vi "Try fsync.vi"(6 "Deadline in":T2, 8 "error in (no error)":errorcluster, 10 "handle":T1 format="%02x", 11 "session in":refnum<class "Session.lvclass">) -> (0 "error out":errorcluster, 3 "session out":refnum<class "Session.lvclass">)   [LabVIEW 2020, in "NI_SFTP.lvlib"]
uses:
  <vilib>/net/SFTP/NI_SFTP.lvlib
  <vilib>/Utility/Deadline/Deadline.ctl
  <vilib>/Utility/Deadline/Mode.ctl
  <vilib>/net/SFTP/Session/Session.lvclass
  <vilib>/net/SFTP/Session/Handle.ctl
  <vilib>/net/SFTP/API/Support/Command/fsync_openssh.com/fsync_openssh.com.lvclass
  <vilib>/Utility/Deadline/NI_Deadline.lvlib
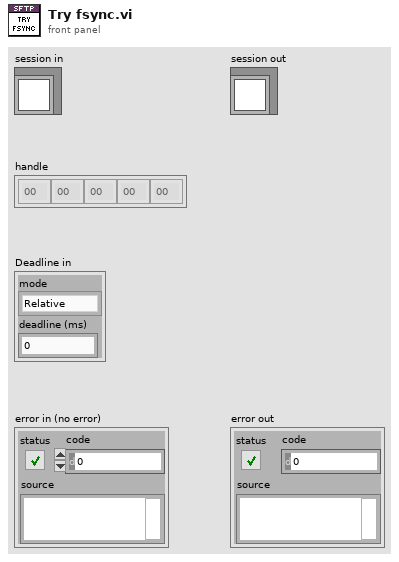
[diagram p1: front panel]
types:
  T1 = typedef "NI_SFTP.lvlib/Session.lvclass/Handle.ctl" = u8[]
  T2 = typedef "NI_Deadline.lvlib/Deadline.ctl" = cluster{"mode":T3, "deadline (ms)":u32}
  T3 = typedef "NI_Deadline.lvlib/Mode.ctl" = enum16{"Relative", "Use deadline", "Wait forever", "Nonblocking", "N/A"}
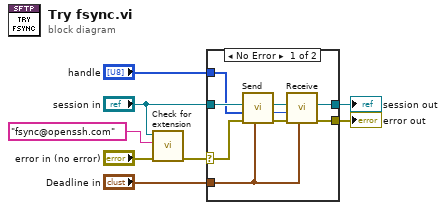
[diagram p0: block diagram]
diagram:
  n1 = call <vilib>:"Check for extension.vi"("error in (no error)"="error in (no error)", "extension name"="fsync@openssh.com" ("name"), "session in"="session in") -> ("error out"=w2:errorcluster)  [unwired: 8 in]
  n2 = case shown="No Error" w2 {
    selector: w2 -> [w14 w18]
    tunnel: "Deadline in" -> [w13 _]
    tunnel: [w17 w18] -> w7
    tunnel: [w9 w19] -> w1
    tunnel: "handle" -> [w11 _]
    tunnel: "session in" -> [w12 w19]
    frame No Error {
      n3 = call <vilib>:"Send.vi"("Timeout"=w13, "error in (no error)"=w14, "handle"=w11, "session in"=w12) -> ("error out"=w16:errorcluster, "request id"=w10:u32, "session out"=w15:refnum<class "Session.lvclass">)  [unwired: 4 in, 1 out]
      n4 = call <vilib>:"Receive.vi"("Timeout"=w13, "error in (no error)"=w16, "request id"=w10, "session in"=w15) -> ("error out"=w17:errorcluster, "session out"=w9:refnum<class "Session.lvclass">)  [unwired: 4 in, 2 out]
    }
    frame Error {
    }
  }
  "error out" <- w7
  "session out" <- w1
